vi "Get Priority.vi"(11 "Timing in":refnum<class "Timing.lvclass">) -> (2 "Priority":u16, 3 "Timing out":refnum<class "Timing.lvclass">)   [LabVIEW 2021, in "DSF Core.lvlib" / "Timing.lvclass"]
uses:
  Timing.lvclass
  Timing.lvclass/Timing.ctl
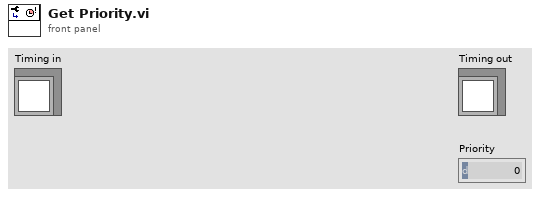
[diagram p1: front panel]
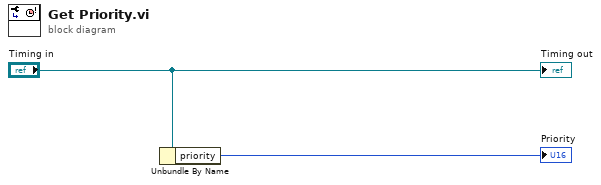
[diagram p0: block diagram]
diagram:
  n1 = Unbundle By Name("Timing in") -> ("priority"=→"Priority":u16)
  "Timing out" <- "Timing in"
